vi "Newest Value Index.vi"(10 "Size":i32, 11 "Index":i32) -> (3 "Newest value index":i32)   [LabVIEW 2021, in "Ring Buffer Time Series Data.lvlib"]
uses:
  Ring Buffer Time Series Data.lvlib
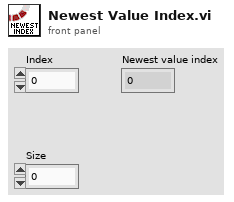
[diagram p1: front panel]
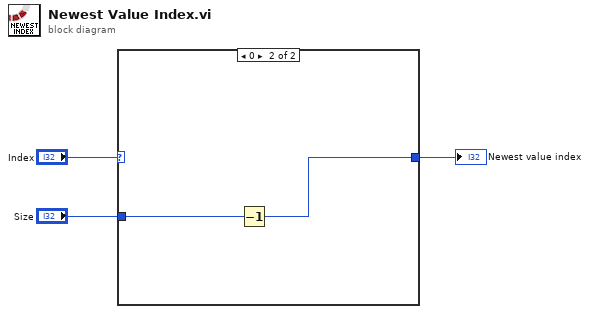
[diagram p0: block diagram]
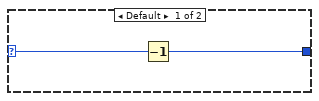
[diagram p2: hidden frame]
diagram:
  n1 = case shown="0" "Index" {
    selector: "Index" -> [w5 _]
    tunnel: [w4 w6] -> w2
    tunnel: "Size" -> [_ w7]
    frame Default {
      n2 = Decrement(x=w5) -> (x-1=w4:i32)
    }
    frame 0 {
      n3 = Decrement(x=w7) -> (x-1=w6:i32)
    }
  }
  "Newest value index" <- w2
